vi "Exercise_3-6_Liam_Hubbard.vi"() -> ()   [LabVIEW 2014]
panel:
  in  "Enum":enum16{"C", "F"}(ring)
  in  "stop":bool
  out "Kelvin":dbl
  out "Celsius":dbl
  out "Farenheit":dbl
  in  "Value":dbl
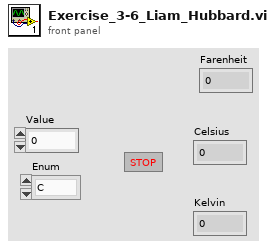
[diagram p1: front panel]
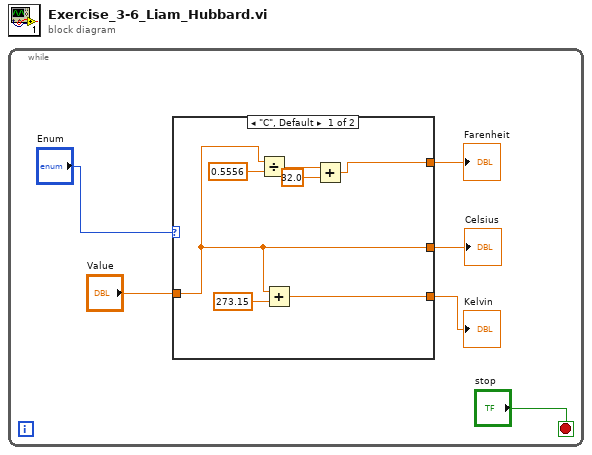
[diagram p0: block diagram]
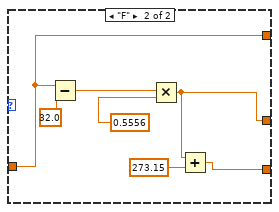
[diagram p2: hidden frame]
diagram:
  n1 = while {
    stop <- "stop" stop-if-true
    n2 = case shown="\"C\", Default" "Enum" {
      tunnel: [w11 w18] -> w6
      tunnel: "Value" -> [w7 w18]
      tunnel: [w7 w15] -> w4
      tunnel: [w9 w16] -> w3
      frame "C", Default {
        n3 = Divide(x=w7, y=0.5556) -> (x/y=w12:dbl)
        n4 = Add(x=w7, y=273.15) -> (x+y=w9:dbl)
        n5 = Add(x=w12, y=32.0) -> (x+y=w11:dbl)
      }
      frame "F" {
        n6 = Subtract(x=w18, y=32.0) -> (x-y=w19:dbl)
        n7 = Multiply(x=w19, y=0.5556) -> (x*y=w15:dbl)
        n8 = Add(x=w15, y=273.15) -> (x+y=w16:dbl)
      }
    }
    "Farenheit" <- w6
    "Celsius" <- w4
    "Kelvin" <- w3
  }
